vi "Input Com Settings.vi"(5 "Serial Port Available?":bool=TRUE, 7 "GEA2 HyperData":bool=TRUE, 9 "COM Port":refnum<visa-resource-name>="COM3") -> (6 "Serial Port Available? Out":bool=TRUE, 8 "GEA2 HyperData Out":bool, 10 "COM Port Out":refnum<visa-resource-name>="COM3")   [LabVIEW 2009]
panel:
  in  "Complete":bool
  # "Communication Setup"
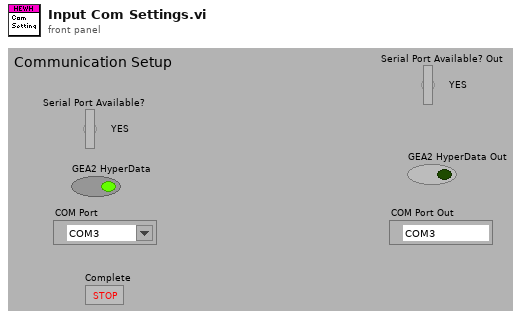
[diagram p1: front panel]
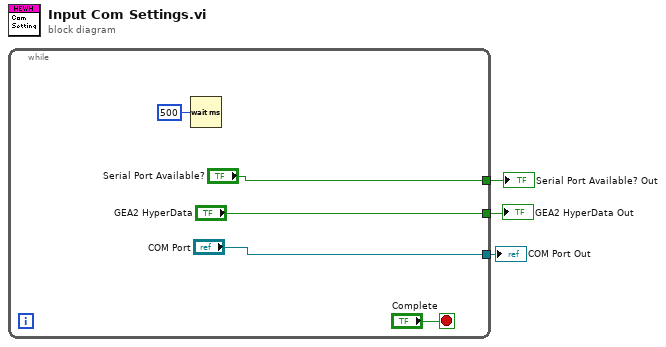
[diagram p0: block diagram]
diagram:
  n1 = while {
    tunnel: ["Serial Port Available?"] -> w3
    tunnel: ["GEA2 HyperData"] -> w2
    tunnel: ["COM Port"] -> w1
    stop <- "Complete" stop-if-true
    n2 = Wait (ms)(milliseconds to wait=u32 500) -> ()  [unwired: 1 out]
  }
  "COM Port Out" <- w1
  "Serial Port Available? Out" <- w3
  "GEA2 HyperData Out" <- w2
